vi "Begin Array.vi"   [LabVIEW 2018, in "Toolkit.lvlib" / "Writer.lvclass"]
doc: "Starts writing and encoding an array to the MessagePack binary data format."
uses:
  Writer.lvclass
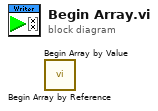
[diagram p0: block diagram]
diagram:
  n1 = call "Begin Array by Reference.vi"() -> ()  [unwired: 10 in, 2 out]
  n2 = call "Begin Array by Value.vi"() -> ()  [unwired: 10 in, 2 out]
